vi "leebinario_carpeta.vi"() -> ()   [LabVIEW 2015]
panel:
  out "size(s)":i32
  out "Waveform Graph 2":sgl[][](graph)
  out "All Files in Dir":path[](array[path])
  out "T, v, UT":sgl[][](array[numeric])
  out "Waveform Graph":waveform(sgl)[](graph)
  out "Array":sgl[][](array[numeric])
  in  "Folder Path":path
  out "error out":errorcluster
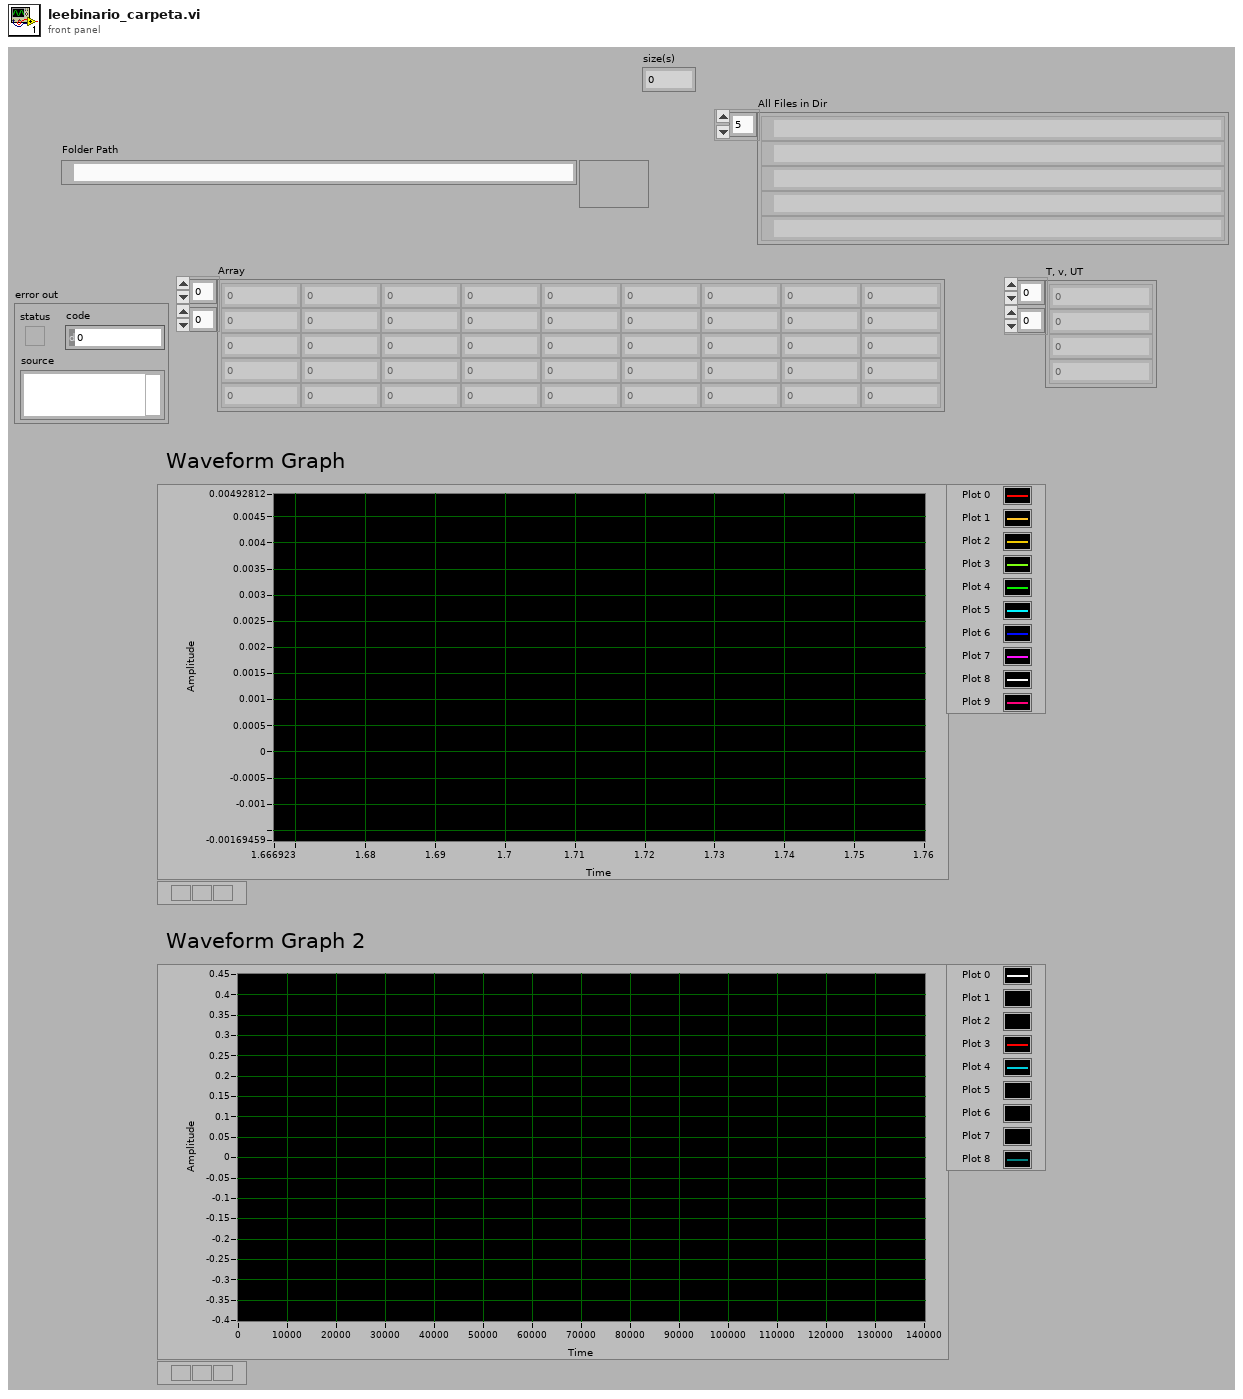
[diagram p1: front panel]
types:
  T1 = enum16{"big-endian, network order", "native, host order", "little-endian"}
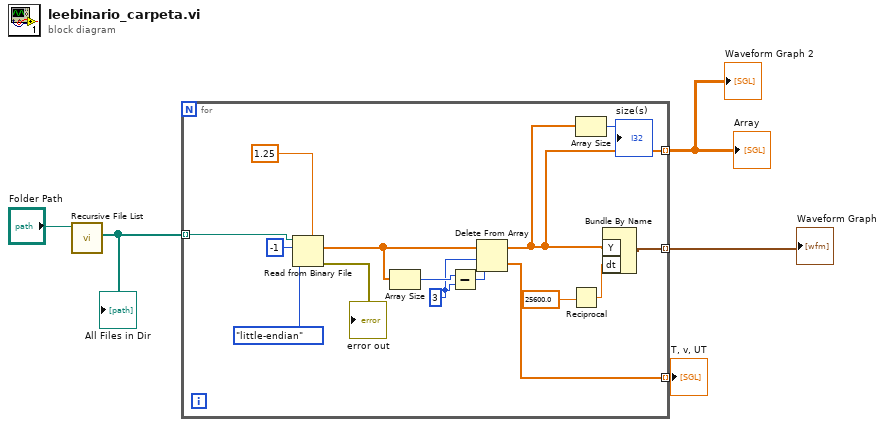
[diagram p0: block diagram]
diagram:
  n1 = call <vilib>:"Recursive File List.vi"("Folder Path"="Folder Path") -> ("All Files in Dir"=w5:path[])  [unwired: 6 in, 4 out]
  "All Files in Dir" <- w5
  n2 = for {
    tunnel: w5 -> [w16] mode=indexing
    tunnel: [w11] -> w3 mode=indexing
    tunnel: [w8] -> w1 mode=indexing
    tunnel: [w6] -> w2 mode=indexing
    w13 = 3 ("length")
    n3 = Read from Binary File(5:sgl 1.25, 9:T1."little-endian" ("byte order (0:big-endian, network order)"), 10:-1 ("count (1)"), 11:w16) -> (0:→"error out":errorcluster, 2:w12:sgl[])  [unwired: 1 in, 3 out]
    n4 = Array Size(array=w12) -> (size(s)=w15:i32)
    n5 = Subtract(x=w15, y=w13) -> (x-y=w14:i32)
    n6 = Delete From Array(array=w12, length=w13, index=w14) -> (deleted portion=w11:sgl[], array with subset deleted=w6:sgl[])
    n7 = Reciprocal(x=25600.0 ("dt")) -> (1/x=w9:dbl)
    n8 = Array Size(array=w6) -> (size(s)=→"size(s)":i32)
    n9 = Bundle By Name("Y"=w6, "dt"=w9) -> (w8:waveform(sgl))  [unwired: 1 in]
  }
  "Array" <- w2
  "Waveform Graph" <- w1
  "T, v, UT" <- w3
  "Waveform Graph 2" <- w2
